vi "frame de minu.vi"() -> ()   [LabVIEW 2021]
uses:
  <vilib>/Instr/_visa.llb/VISA Configure Serial Port (Instr).vi
panel:
  out "String 2":string
  in  "VISA resource name":refnum<visa-resource-name>
  in  "REFRESH":bool
  out "Thermometer":dbl(slide) scale=0.0..100.0
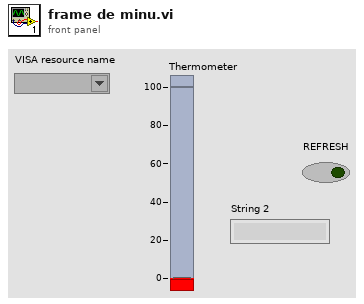
[diagram p1: front panel]
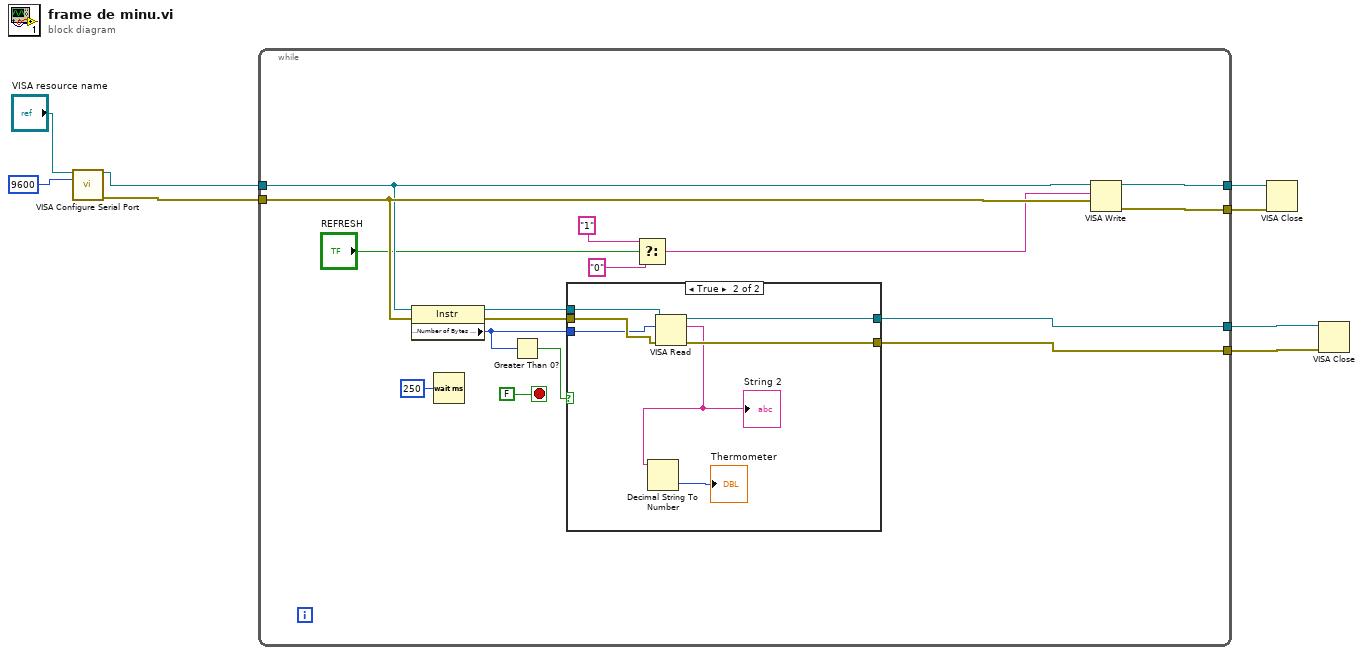
[diagram p0: block diagram]
diagram:
  n1 = call-poly "VISA Configure Serial Port"("VISA resource name"="VISA resource name", "baud rate (9600)"=u32 9600) -> ("VISA resource name out"=w8:refnum<visa-resource-name>, "error out"=w6:errorcluster)  [unwired: 12 in]
  n2 = while {
    tunnel: w8 -> [w14]
    tunnel: [w24] -> w7
    tunnel: w6 -> [w15]
    tunnel: [w23] -> w5
    tunnel: [w20] -> w2
    tunnel: [w19] -> w1
    stop <- FALSE stop-if-true
    n3 = property class="Instr"(reference=w14, error in=w15) -> (reference out=w18:refnum<visa-resource-name>, error out=w13:errorcluster, "Serial Settings:Number of Bytes at Serial Port"=w9:u32)
    n4 = Wait (ms)(milliseconds to wait=u32 250) -> ()  [unwired: 1 out]
    n5 = Greater Than 0?(x=w9) -> (x > 0?=w10:bool)
    n6 = case shown="True" w10 {
      tunnel: [w26 w33] -> w20
      tunnel: [w25 w32] -> w19
      tunnel: w18 -> [w26 w31]
      tunnel: w13 -> [w25 w30]
      tunnel: w9 -> [_ w27]
      frame False {
      }
      frame True {
        n7 = VISA Read(VISA resource name=w31, byte count=w27, error in (no error)=w30) -> (VISA resource name out=w33:refnum<visa-resource-name>, read buffer=w28:string, error out=w32:errorcluster)  [unwired: 1 out]
        "String 2" <- w28
        n8 = Decimal String To Number(string=w28) -> (number=→"Thermometer":i32)  [unwired: 2 in, 1 out]
      }
    }
    n9 = Select(t="1", s="REFRESH", f="0") -> (s? t:f=w12:string)
    n10 = VISA Write(VISA resource name=w14, write buffer=w12, error in (no error)=w15) -> (VISA resource name out=w24:refnum<visa-resource-name>, error out=w23:errorcluster)  [unwired: 1 out]
  }
  n11 = VISA Close(VISA resource name=w7, error in (no error)=w5) -> ()  [unwired: 1 out]
  n12 = VISA Close(VISA resource name=w2, error in (no error)=w1) -> ()  [unwired: 1 out]
